vi "Hopper Calibration.vi"(9 "Boolean":bool) -> ()   [LabVIEW 2012]
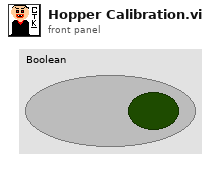
[diagram p1: front panel]
types:
  T1 = typedef "WPI_DigitalInputDevRef.ctl" = cluster{"DevStatus":errorcluster, "DIO Channel":T2, "Digital Module":T3}
  T2 = typedef "FPGA_DIOChannel.ctl" = enum8{"DIO 1", "DIO 2", "DIO 3", "DIO 4", "DIO 5", "DIO 6", "DIO 7", "DIO 8", "DIO 9", "DIO 10", "DIO 11", "DIO 12", "DIO 13", "DIO 14", "Invalid"}
  T3 = typedef "FPGA_TypedefDigitalModule.ctl" = enum16{"Digital Module 1", "Digital Module 2"}
  T4 = typedef "WPI_MotorControlDeviceRef.ctl" = cluster{"DeviceStatus":errorcluster, "Type":enum16{"PWM", "CAN"}, "PWM":cluster{"Digital Module":T3, "PWM Channel":T5, "DeadBand":T6}, "CAN":cluster{"Device Number":u8, "Control Mode":T7, "Semaphore":T8, "Max Vout":dbl}, "Invert":bool, "TransformRef":T9, "InvTransformRef":T9}
  T5 = typedef "FPGA_DIOPWMChannel.ctl" = enum8{"PWM 1", "PWM 2", "PWM 3", "PWM 4", "PWM 5", "PWM 6", "PWM 7", "PWM 8", "PWM 9", "PWM 10", "Invalid"}
  T6 = typedef "WPI_PWMDeadband.ctl" = cluster{"Name":string, "maxPositivePwm":i32, "minPositivePwm":i32, "centerPwm":i32, "maxNegativePwm":i32, "minNegativePwm":i32, "angularRange":u16}
  T7 = typedef "WPI_CANJaguar_ControlMode.ctl" = enum8{"Percent VBus", "Current", "Speed", "Position", "Voltage"}
  T8 = typedef "Semaphore RefNum" = refnum<k1>
  T9 = typedef "WPI_PWMTransform_ConPane.ctl" = refnum<vi>
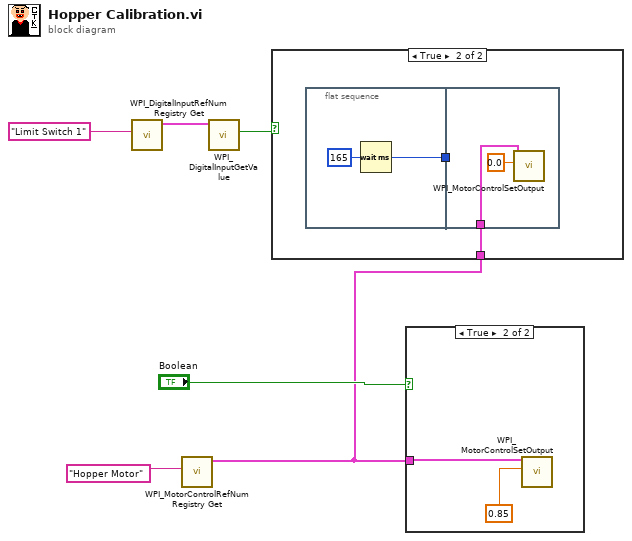
[diagram p0: block diagram]
diagram:
  n1 = call <vilib>:"WPI_DigitalInputRefNum Registry Get.vi"("refnum name"="Limit Switch 1") -> ("DigitalInputDevRef"=w3:T1)  [unwired: 9 in, 1 out]
  n2 = call <vilib>:"WPI_MotorControlRefNum Registry Get.vi"("refnum name"="Hopper Motor") -> ("MotorControlDevRef"=w1:T4)  [unwired: 9 in, 1 out]
  n3 = call <vilib>:"WPI_DigitalInputGetValue.vi"("DigitalInputDevRef"=w3) -> ("Value"=w2:bool)  [unwired: 8 in, 2 out]
  n4 = case shown="True" w2 {
    tunnel: w1 -> [_ w7]
    frame False {
    }
    frame True {
      n5 = flat-sequence {
        tunnel: [w9] -> w8
        tunnel: w8 -> [_]
        tunnel: w7 -> [w12]
        frame #0 {
          n6 = Wait (ms)(milliseconds to wait=u32 165) -> (millisecond timer value=w9:u32)
        }
        frame #1 {
          n7 = call <vilib>:"WPI_MotorControlSetOutput.vi"("Output"=0.0, "MotorControlDevRef"=w12) -> ()  [unwired: 7 in, 3 out]
        }
      }
    }
  }
  n8 = case shown="True" "Boolean" {
    tunnel: w1 -> [_ w13]
    frame False {
    }
    frame True {
      n9 = call <vilib>:"WPI_MotorControlSetOutput.vi"("Output"=0.85, "MotorControlDevRef"=w13) -> ()  [unwired: 7 in, 3 out]
    }
  }
